vi "UHR-Fleezers Control (host) -Leonardo 04-2018 V3_greenctrl.vi"(0 "Tab Green FB":T5(tab)=enum."Trap Control (RF)") -> ()   [LabVIEW 2013] (continued)
        n482 = property on="APD Chart" class="WFChart (strict)"("YScale.Minimum"=w832) -> ()  [unwired: 2 in, 2 out]
        n483 = property on="APD Chart" class="WFChart (strict)"("YScale.Maximum"=w831) -> ()  [unwired: 2 in, 2 out]
      }
      event "Phase adj. (AI1)", "+ phase (AI1)", "- phase (AI1)": Value Change {
        n484 = event-data() -> ()  [unwired: 7 out]
        n485 = Negate(x="Phase adj. (AI1)") -> (-x=w848:i16)
        n486 = Select(t=w848, s="- phase (AI1)", f="Phase adj. (AI1)") -> (s? t:f=w847:i16)
        n487 = xnode "Read/Write Control"("FPGA VI Reference In"=w851, "error in"=w850, "Phase count adjustment"=w847) -> ("FPGA VI Reference Out"=w846:T20, "error out"=w845:errorcluster)
        n488 = Or(x="- phase (AI1)", y="+ phase (AI1)") -> (x .or. y?=w842:bool)
        n489 = xnode "Read/Write Control"("FPGA VI Reference In"=w846, "error in"=w845, "+ phase"=w842) -> ("error out"=w841:errorcluster)  [unwired: 1 out]
      }
      event "Signals to Plot": Double Click {
        w854 = u32 9868950 ("Color Box")
        n490 = event-data() -> ("Row"=w856:i32)  [unwired: 9 out]
        n491 = property on="All Signals" class="WFChart (strict)"("Active Plot"=w856) -> (error out=w867:errorcluster)  [unwired: 2 in, 1 out]
        n492 = property on="All Signals" class="WFChart (strict)" props=["Plot", "Visible?", "Plot", "Plot Color"](error in=w867) -> (error out=w866:errorcluster, "Plot.Visible?"=w865:bool)  [unwired: 1 in, 2 out]
        n493 = Select(t=FALSE ("Plot.Visible"), s=w865, f=TRUE ("Plot.Visible")) -> (s? t:f=w860:bool)
        n494 = property on="All Signals" class="WFChart (strict)"(error in=w866, "Plot.Visible?"=w860) -> (error out=w862:errorcluster)  [unwired: 1 in, 1 out]
        n495 = property on="All Signals" class="WFChart (strict)"(error in=w862) -> (error out=w857:errorcluster, "Plot.Plot Color"=w861:u32)  [unwired: 1 in, 1 out]
        n496 = property on="Signals to Plot" class="LstBox (strict)"(error in=w857, "Active Row"=w856) -> (error out=w855:errorcluster)  [unwired: 1 in, 1 out]
        n497 = Select(t=w861, s=w860, f=u32 0) -> (s? t:f=w858:u32)
        n498 = property on="Signals to Plot" class="LstBox (strict)"(error in=w855, "CellFontColor"=w858, "SelColor"=w854, "CellBG"=w854, "CellFontSize"=u32 20 ("Active Row:Cell Font:Size"), "CellFontBold"=TRUE ("Active Row:Cell Font:Bold")) -> ()  [unwired: 1 in, 2 out]
      }
      event "Dynamic Force FB": Value Change {
        n499 = event-data() -> ()  [unwired: 7 out]
        n500 = xnode "Read/Write Control"("FPGA VI Reference In"=w869, "Dynamic Force FB (Ronen)"="Dynamic Force FB") -> ()  [unwired: 1 in, 2 out]
      }
      event "BD 1 Frequency 1 (MHz)", "BD 1 Frequency 2 (MHz)", "BD 1 Frequency 3 (MHz)", "BD 2 Frequency 1 (MHz)", "BD 2 Frequency 2 (MHz)", "BD 2 Frequency 3 (MHz)", "Trap Delta (MHz)": Value Change {
        # "anytime one of the frequencies is changed, write it to the RF board UNLESS Set 2 is being oscillated. The oscillation\nscript writes the frequencies to the RF board."
        n501 = event-data() -> ("CtlRef"=w872:refnum<vi>)  [unwired: 6 out]
        n502 = control-ref of="Trap Delta (MHz)"() -> (w871:refnum<vi>)
        n503 = Equal?(x=w871, y=w872) -> (x = y?=w870:bool)
        n504 = case shown="False" "Oscillate Set 2" {
          tunnel: w875 -> [w896 _]
          tunnel: [w895 w908] -> w874
          tunnel: w873 -> [w894 w908]
          tunnel: w870 -> [w881 _]
          frame False {
            n505 = case shown="True" "Symmetric manual \ntrap motion" {
              tunnel: ["T2 for asymmetric\n(MHz)" w907] -> w882
              tunnel: "Trap Delta (MHz)" -> [w901 w906]
              tunnel: [w900 w903] -> w878
              frame False {
                n506 = Subtract(x="T2 for asymmetric\n(MHz)", y=w901) -> (x-y=w900:dbl)
              }
              frame True {
                n507 = Divide(x=w906, y=2) -> (x/y=w904:dbl)
                n508 = Subtract(x="Middle freq for \nsymmetric (MHz)", y=w904) -> (x-y=w903:dbl)
                n509 = Add(x="Middle freq for \nsymmetric (MHz)", y=w904) -> (x+y=w907:dbl)
              }
            }
            n510 = local read "BD 1 Frequency 2 (MHz)"() -> (w883:dbl)
            n511 = local write "BD 1 Frequency 1 (MHz)"(w878) -> ()
            n512 = Select(t=w882, s=w881, f=w883) -> (s? t:f=w880:dbl)
            n513 = local read "Y RF Frequency Limits (MHz)"() -> (w884:T16)
            n514 = local read "X RF Frequency Limits (MHz)"() -> (w885:T16)
            n515 = local read "BD 1 Frequency 3 (MHz)"() -> (w897:dbl)
            n516 = local write "BD 1 Frequency 2 (MHz)"(w880) -> ()
            n517 = local read "BD 2 Frequency 1 (MHz)"() -> (w888:dbl)
            n518 = local read "BD 2 Frequency 2 (MHz)"() -> (w887:dbl)
            n519 = local read "BD 2 Frequency 3 (MHz)"() -> (w898:dbl)
            n520 = call "set RF board frequency - interlace.vi"("Board 2 Frequency Limits"=w884, "Board 1 Frequency Limits"=w885, "error in"=w894, "FPGA VI Reference In"=w896, "Board 2 Frequency 3 (MHz)"=w898, "Board 1 Frequency 3 (MHz)"=w897, "Board 2 Frequency 2 (MHz)"=w887, "Board 2 Frequency 1 (MHz)"=w888, "Board 1 Frequency 2 (MHz)"=w880, "Board 1 Frequency 1  (MHz)"=w878) -> ("error out"=w895:errorcluster)  [unwired: 1 out]
            n521 = Subtract(x=w888, y=w887) -> (x-y=w892:dbl)
            n522 = Subtract(x=w880, y=w878) -> (x-y=w893:dbl)
            n523 = Square(x=w892) -> (x^2=w890:dbl)
            n524 = Square(x=w893) -> (x^2=w891:dbl)
            n525 = Add(x=w891, y=w890) -> (x+y=w889:dbl)
            n526 = Square Root(x=w889) -> (sqrt(x)=w886:dbl)
            n527 = local write "Trap Delta (MHz)"(w886) -> ()
            n528 = property on="Initial delta (MHz)" class="DigNum (strict)"("Val(Sgnl)"=w886) -> ()  [unwired: 2 in, 2 out]
          }
          frame True {
          }
        }
      }
      event "Round T1 X": Value Change {
        n529 = event-data() -> ()  [unwired: 7 out]
        n530 = local read "BD 1 Frequency 1 (MHz)"() -> (w911:dbl)
        n531 = Round To Nearest(number=w911) -> (nearest integer value=w910:dbl)
        n532 = property on="BD 1 Frequency 1 (MHz)" class="DigNum (strict)"("Val(Sgnl)"=w910) -> ()  [unwired: 2 in, 2 out]
      }
      event "Round T2 X": Value Change {
        n533 = event-data() -> ()  [unwired: 7 out]
        n534 = local read "BD 1 Frequency 2 (MHz)"() -> (w913:dbl)
        n535 = Round To Nearest(number=w913) -> (nearest integer value=w912:dbl)
        n536 = property on="BD 1 Frequency 2 (MHz)" class="DigNum (strict)"("Val(Sgnl)"=w912) -> ()  [unwired: 2 in, 2 out]
      }
      event "Stop All": Value Change {
        n537 = event-data() -> ()  [unwired: 7 out]
        n538 = call "hamilton_controller.vi"("action"=T21."DISCONNECT") -> ()  [unwired: 10 in, 1 out]
        n539 = local read "Stop All"() -> (w916:bool)
      }
      event "Delayed Interlace Start": Value Change {
        n540 = event-data() -> ()  [unwired: 7 out]
        n541 = flat-sequence {
          frame #0 {
            n542 = Multiply(x="Delay to Interlace (s)", y=1000.0) -> (x*y=w919:dbl)
            n543 = Wait (ms)(milliseconds to wait=w919) -> ()  [unwired: 1 out]
          }
          frame #1 {
            n544 = property on="Green laser mode" class="RadioBtnsControl (strict)"("Val(Sgnl)"=enum32{"Laser ON", "Laser OFF", "Interlace"}."Interlace" ("Value (Signaling)")) -> ()  [unwired: 2 in, 2 out]
          }
        }
      }
      event "BD 1 Amplitude 1 (%)", "BD 1 Amplitude 2 (%)", "BD 1 Amplitude 3 (%)", "BD 2 Amplitude 1 (%)", "BD 2 Amplitude 2 (%)", "BD 2 Amplitude 3 (%)", "Trap 1 ON", "Trap 2 ON", "Trap 3 ON", "Feedback On/Off", "All FB On/Off": Value Change {
        w943 = i16 1 ("f")
        n545 = event-data() -> ()  [unwired: 7 out]
        n546 = local write "Trap 1 (ON/OFF)"("Trap 1 ON") -> ()
        n547 = local write "Trap 2 (ON/OFF)"("Trap 2 ON") -> ()
        n548 = Boolean To (0,1)(Boolean="Trap 3 ON") -> (0, 1=w944:i16)
        n549 = Boolean To (0,1)(Boolean="Trap 1 ON") -> (0, 1=w945:i16)
        n550 = Boolean To (0,1)(Boolean="Trap 2 ON") -> (0, 1=w946:i16)
        n551 = Select(t=w946, s="Trap ON/OFF X or Y Amp?", f=w943) -> (s? t:f=w941:i16)
        n552 = Select(t=w945, s="Trap ON/OFF X or Y Amp?", f=w943) -> (s? t:f=w942:i16)
        n553 = Select(t=w944, s="Trap ON/OFF X or Y Amp?", f=w943) -> (s? t:f=w940:i16)
        n554 = Select(t=w943, s="Trap ON/OFF X or Y Amp?", f=w946) -> (s? t:f=w938:i16)
        n555 = Select(t=w943, s="Trap ON/OFF X or Y Amp?", f=w945) -> (s? t:f=w939:i16)
        n556 = Select(t=w943, s="Trap ON/OFF X or Y Amp?", f=w944) -> (s? t:f=w937:i16)
        n557 = And(x="All FB On/Off", y="Feedback On/Off") -> (x .and. y?=w935:cluster{"Set 1":bool, "Set 2":bool})
        n558 = local read "BD 1 Amplitude 1 (%)"() -> (w955:dbl)
        n559 = local read "BD 1 Amplitude 2 (%)"() -> (w954:dbl)
        n560 = local read "BD 1 Amplitude 3 (%)"() -> (w953:dbl)
        n561 = Unbundle By Name(w935) -> ("Set 1"=w931:bool, "Set 2"=w928:bool)
        n562 = local read "Y RF Amplitude Limits (%)"() -> (w924:T16)
        n563 = local read "X RF Amplitude Limits (%)"() -> (w925:T16)
        n564 = local read "BD 2 Amplitude 1 (%)"() -> (w956:dbl)
        n565 = local read "BD 2 Amplitude 2 (%)"() -> (w957:dbl)
        n566 = local read "BD 2 Amplitude 3 (%)"() -> (w958:dbl)
        n567 = And(x="Trap 2 ON", y=w928) -> (x .and. y?=w926:bool)
        n568 = And(x="Trap 1 ON", y=w931) -> (x .and. y?=w929:bool)
        n569 = Multiply(x=w942, y=w955) -> (x*y=w950:dbl)
        n570 = Multiply(x=w954, y=w941) -> (x*y=w948:dbl)
        n571 = Multiply(x=w953, y=w940) -> (x*y=w949:dbl)
        n572 = Multiply(x=w956, y=w939) -> (x*y=w959:dbl)
        n573 = Multiply(x=w957, y=w938) -> (x*y=w960:dbl)
        n574 = Multiply(x=w958, y=w937) -> (x*y=w961:dbl)
        n575 = call "set RF board amplitude - interlace.vi"("Board 2 Amplitude Limits"=w924, "Board 1 Amplitude Limits"=w925, "error in"=w951, "FPGA VI Reference In"=w952, "Board 2 Amplitude 3 (%)"=w961, "Board 1 Amplitude 3 (%)"=w949, "Board 2 Amplitude 2 (%)"=w960, "Board 2 Amplitude 1 (%)"=w959, "Board 1 Amplitude 2 (%)"=w948, "Board 1 Amplitude 1 (%)"=w950) -> ("error out"=w933:errorcluster, "FPGA VI Reference Out"=w934:T20)
        n576 = xnode "Read/Write Control"("FPGA VI Reference In"=w934, "error in"=w933, "FB On/Off Set 1"=w929, "FB On/Off Set 2"=w926) -> ("error out"=w932:errorcluster)  [unwired: 1 out]
        n577 = case shown="True" "All FB On/Off" {
          frame False {
          }
          frame True {
            n578 = local write "Feedback overload"(FALSE) -> ()
          }
        }
      }
      event "Load parameters": Value Change {
        n579 = event-data() -> ()  [unwired: 7 out]
        n580 = property on="Saved AOD Raster Scan Parameter Sets" class="Arr (strict)"() -> ("Index Values"=w973:u32[])  [unwired: 2 in, 2 out]
        n581 = Index Array(array=w973, index=0) -> (element=w970:u32)
        n582 = local write "Load parameters"(FALSE ("Load parameters")) -> ()
        n583 = Index Array(array="Saved AOD Raster Scan Parameter Sets", index=w970) -> (element=w969:T31)
        n584 = Unbundle By Name(w969) -> ("Scan Range AOD (nm) 2"=w968:dbl, "Step Size AOD (nm) 2"=w967:dbl, "Scan Speed AOD (nm/s) 2"=w966:dbl, "Number of scans (AOD) 2"=w965:u16)
        n585 = flat-sequence {
          tunnel: w968 -> [w976]
          tunnel: w967 -> [w975]
          tunnel: w966 -> [w974]
          tunnel: w965 -> [w977]
          frame #0 {
            n586 = local write "Scan Speed (nm/s)"(w974) -> ()
            n587 = local write "Scan Range (nm)"(w976) -> ()
            n588 = local write "Step Size (nm)"(w975) -> ()
          }
          frame #1 {
            n589 = property on="Number of F/B Scans (AOD)" class="DigNum (strict)"("Val(Sgnl)"=w977) -> ()  [unwired: 2 in, 2 out]
          }
        }
      }
      event "Trap 1 (ON/OFF)", "Trap 2 (ON/OFF)": Value Change {
        n590 = event-data() -> ()  [unwired: 7 out]
        n591 = property on="Trap 2 ON" class="Bool (strict)"("Val(Sgnl)"="Trap 2 (ON/OFF)") -> ()  [unwired: 2 in, 2 out]
        n592 = property on="Trap 1 ON" class="Bool (strict)"("Val(Sgnl)"="Trap 1 (ON/OFF)") -> ()  [unwired: 2 in, 2 out]
      }
      event "DIO count 1 (ticks)", "DIO count 2 (ticks)", "DIO count 3 (ticks)", "Interlace", "Number Interlace Sets", "Not-Interlacing Set": Value Change {
        n593 = event-data() -> ()  [unwired: 7 out]
        n594 = local read "DIO count 3 (ticks)"() -> (w990:u32)
        n595 = local read "DIO count 1 (ticks)"() -> (w992:u32)
        n596 = local read "DIO count 2 (ticks)"() -> (w991:u32)
        n597 = To Unsigned Byte Integer(number="Not-Interlacing Set") -> (unsigned 8bit integer=w981:u8)
        n598 = Add(x=w981, y=u8 1) -> (x+y=w985:u8)
        n599 = xnode "Read/Write Control"("FPGA VI Reference In"=w996, "error in"=w994, "DIO count 1 (ticks)"=w992, "DIO count 2 (ticks)"=w991, "DIO count 3 (ticks)"=w990, "Interlace ON/OFF"="Interlace", "Number Interlace Cycles"="Number Interlace Sets", "Interlace Off Parameters"=w985) -> ("error out"=w995:errorcluster)  [unwired: 1 out]
        n600 = Build Array(w992, w991, w990) -> (w983:u32[])
        n601 = Split 1D Array(array=w983, index="Number Interlace Sets") -> (first subarray=w993:u32[])  [unwired: 1 out]
        n602 = Index Array(array=w983, index=w981) -> (element=w982:u32)
        n603 = Add Array Elements(numeric array=w993) -> (sum=w987:u32)
        n604 = Select(t=w987, s="Interlace", f=w982) -> (s? t:f=→"Total Counts (ticks)":u32)
      }
      event "Reset Feedback": Value Change {
        n605 = event-data() -> ()  [unwired: 7 out]
        n606 = Unbundle By Name("Reset Feedback") -> ("Set 1"=w1000:bool, "Set 2"=w999:bool)
        n607 = xnode "Read/Write Control"("FPGA VI Reference In"=w1002, "error in"=w997, "FB Reset Set 1"=w1000, "FB Reset Set 2"=w999) -> ("error out"=w998:errorcluster)  [unwired: 1 out]
      }
      event "PID gains": Value Change {
        n608 = event-data() -> ()  [unwired: 7 out]
        n609 = local read "PID gains"() -> (w1003:T10)
        n610 = xnode "Read/Write Control"("FPGA VI Reference In"=w1006, "error in"=w1004, "FB Gains"=w1003) -> ("error out"=w1005:errorcluster)  [unwired: 1 out]
      }
      event "AI2 to Setpoint", "Trap Intensity\nSetpoints (V)": Value Change {
        n611 = event-data() -> ()  [unwired: 7 out]
        n612 = xnode "Read/Write Control"("FPGA VI Reference In"=w1011, "error in"=w1007) -> ("FPGA VI Reference Out"=w1010:T20, "error out"=w1009:errorcluster, "AI2 Y Sum Set 1"=w1018:i16, "AI2 Y Sum Set 2"=w1017:i16)
        n613 = Cluster To Array(cluster="AI2 to Setpoint") -> (array=w1021:bool[])
        n614 = local read "AI2 (V)"() -> (w1019:cluster{"Set 1":dbl, "Set 2":dbl})
        n615 = Or Array Elements(Boolean array=w1021) -> (logical OR=w1022:bool)
        n616 = Bundle By Name(cluster=w1019, "Set 1"=w1018, "Set 2"=w1017) -> (w1016:cluster{"Set 1":dbl, "Set 2":dbl})
        n617 = Divide(x=w1016, y=3276.7) -> (x/y=w1015:cluster{"Set 1":dbl, "Set 2":dbl})
        "AI2 (V)" <- w1015
        n618 = case shown="True" w1022 {
          tunnel: [w1025 w1042] -> w1014
          tunnel: "AI2 to Setpoint" -> [_ w1038]
          tunnel: "Trap Intensity\nSetpoints (V)" -> [w1026 w1041]
          tunnel: w1015 -> [_ w1035]
          frame False {
            n619 = Multiply(x=3276.7, y=w1026) -> (x*y=w1027:cluster{"Set 1":dbl, "Set 2":dbl})
            n620 = To Word Integer(number=w1027) -> (16bit integer=w1025:cluster{"Set 1":i16, "Set 2":i16})
          }
          frame True {
            n621 = Unbundle By Name(w1035) -> ("Set 1"=w1034:dbl, "Set 2"=w1033:dbl)
            n622 = Unbundle By Name(w1041) -> ("Set 1"=w1040:dbl, "Set 2"=w1039:dbl)
            n623 = Unbundle By Name(w1038) -> ("Set 1"=w1037:bool, "Set 2"=w1036:bool)
            n624 = Select(t=w1034, s=w1037, f=w1040) -> (s? t:f=w1032:dbl)
            n625 = Select(t=w1033, s=w1036, f=w1039) -> (s? t:f=w1031:dbl)
            n626 = Bundle By Name(cluster=w1041, "Set 1"=w1032, "Set 2"=w1031) -> (w1029:cluster{"Set 1":dbl, "Set 2":dbl})
            n627 = local write "Trap Intensity\nSetpoints (V)"(w1029) -> ()
            n628 = Multiply(x=3276.7, y=w1029) -> (x*y=w1030:cluster{"Set 1":dbl, "Set 2":dbl})
            n629 = To Word Integer(number=w1030) -> (16bit integer=w1042:cluster{"Set 1":i16, "Set 2":i16})
          }
        }
        n630 = Unbundle By Name(w1014) -> ("Set 1"=w1013:i16, "Set 2"=w1012:i16)
        n631 = xnode "Read/Write Control"("FPGA VI Reference In"=w1010, "error in"=w1009, "FB Setpoint Set 1"=w1013, "FB Setpoint Set 2"=w1012) -> ("error out"=w1008:errorcluster)  [unwired: 1 out]
      }
      event "Invert GI": Value Change {
        n632 = event-data() -> ()  [unwired: 7 out]
        n633 = xnode "Read/Write Control"("FPGA VI Reference In"=w1047, "error in"=w1045, "Invert GI"="Invert GI", "Invert GI 2"="Invert GI") -> ("error out"=w1046:errorcluster)  [unwired: 1 out]
      }
      event "Green FB Setpoint (mV)", "Green FB Gains", "Green FB On/Off", "Current When FB OFF (%)", "Green int current ON count adj": Value Change {
        n634 = event-data() -> ()  [unwired: 7 out]
        n635 = local read "Green FB Setpoint (mV)"() -> (w1054:dbl)
        n636 = local read "Current When FB OFF (%)"() -> (w1057:dbl)
        n637 = Multiply(x=w1054, y=3.2767) -> (x*y=w1053:dbl)
        n638 = Multiply(x=w1057, y=655.35) -> (x*y=w1058:dbl)
        n639 = To Unsigned Word Integer(number=w1058) -> (unsigned 16bit integer=w1056:u16)
        n640 = local read "Green int current ON count adj"() -> (w1061:u32)
        n641 = local read "Green FB Gains"() -> (w1060:T10)
        n642 = local read "Green Laser ON/Interlacing"() -> (w1051:bool)
        n643 = local read "Green laser mode"() -> (w1050:enum32{"Laser ON", "Laser OFF", "Interlace"})
        n644 = local read "Green FB On/Off"() -> (w1062:bool)
        n645 = Equal?(x=w1050, y=enum32{"Laser ON", "Laser OFF", "Interlace"}."Interlace") -> (x = y?=w1048:bool)
        n646 = Compound Arithmetic op=AND(w1048, w1062, w1051) -> (w1052:bool)
        n647 = xnode "Read/Write Control"("FPGA VI Reference In"=w1065, "error in"=w1064, "Green FB Setpoint"=w1053, "Green FB On/Off"=w1052, "Current Out"=w1056, "Green int current ON count adj"=w1061, "Green FB Gains"=w1060) -> ("error out"=w1063:errorcluster)  [unwired: 1 out]
      }
      event "Green laser mode", "Green Laser ON/Interlacing": Value Change {
        n648 = event-data() -> ()  [unwired: 7 out]
        n649 = case shown="True" "Green Laser ON/Interlacing" {
          tunnel: "Green laser mode" -> [_ w1079]
          tunnel: [enum32{"Laser ON", "Laser OFF", "Interlace"}."Laser OFF" ("Green laser mode") w1079] -> w1067
          tunnel: [FALSE w1075] -> w1066
          frame False {
          }
          frame True {
            n650 = local read "Green FB On/Off"() -> (w1076:bool)
            n651 = Equal?(x=w1079, y=enum32{"Laser ON", "Laser OFF", "Interlace"}."Interlace") -> (x = y?=w1077:bool)
            n652 = And(x=w1077, y=w1076) -> (x .and. y?=w1075:bool)
          }
        }
        n653 = xnode "Read/Write Control"("FPGA VI Reference In"=w1072, "error in"=w1070, "Operating Mode"=w1067, "Operating Mode 2"=w1067, "Green FB On/Off"=w1066) -> ("error out"=w1071:errorcluster)  [unwired: 1 out]
      }
      event "- phase (APD 1 Gate)", "+ phase (APD 1 Gate)": Value Change {
        n654 = event-data() -> ()  [unwired: 7 out]
        n655 = local read "Phase Adj. (APD 1 Gate)"() -> (w1080:i16)
        n656 = Negate(x=w1080) -> (-x=w1088:i16)
        n657 = Select(t=w1088, s="- phase (APD 1 Gate)", f=w1080) -> (s? t:f=w1087:i16)
        n658 = Or(x="- phase (APD 1 Gate)", y="+ phase (APD 1 Gate)") -> (x .or. y?=w1083:bool)
        n659 = xnode "Read/Write Control"("FPGA VI Reference In"=w1090, "error in"=w1089, "Phase count adjustment (APD 1 Gate)"=w1087) -> ("FPGA VI Reference Out"=w1085:T20, "error out"=w1086:errorcluster)
        n660 = xnode "Read/Write Control"("FPGA VI Reference In"=w1085, "error in"=w1086, "+ phase (APD 1 Gate)"=w1083) -> ("error out"=w1084:errorcluster)  [unwired: 1 out]
      }
      event "+ phase (APD 2 Gate)", "- phase (APD 2 Gate)": Value Change {
        n661 = event-data() -> ()  [unwired: 7 out]
        n662 = local read "Phase Adj. (APD 2 Gate)"() -> (w1091:i16)
        n663 = Negate(x=w1091) -> (-x=w1099:i16)
        n664 = Select(t=w1099, s="- phase (APD 2 Gate)", f=w1091) -> (s? t:f=w1098:i16)
        n665 = Or(x="- phase (APD 2 Gate)", y="+ phase (APD 2 Gate)") -> (x .or. y?=w1094:bool)
        n666 = xnode "Read/Write Control"("FPGA VI Reference In"=w1101, "error in"=w1100, "Phase count adjustment (APD 2 Gate)"=w1098) -> ("FPGA VI Reference Out"=w1096:T20, "error out"=w1097:errorcluster)
        n667 = xnode "Read/Write Control"("FPGA VI Reference In"=w1096, "error in"=w1097, "+ phase (APD 2 Gate)"=w1094) -> ("error out"=w1095:errorcluster)  [unwired: 1 out]
      }
      event "Phase Adj. (APD Acq)", "+ phase (APD Acq)", "- phase (APD Acq)": Value Change {
        n668 = event-data() -> ()  [unwired: 7 out]
        n669 = local read "Phase Adj. (APD Acq)"() -> (w1104:i16)
        n670 = Negate(x=w1104) -> (-x=w1110:i16)
        n671 = Select(t=w1110, s="+ phase (APD Acq)", f=w1104) -> (s? t:f=w1109:i16)
        n672 = Or(x="+ phase (APD Acq)", y="- phase (APD Acq)") -> (x .or. y?=w1105:bool)
        n673 = xnode "Read/Write Control"("FPGA VI Reference In"=w1112, "error in"=w1111, "Phase Count Adjustment (APD Acq)"=w1109) -> ("FPGA VI Reference Out"=w1107:T20, "error out"=w1108:errorcluster)
        n674 = xnode "Read/Write Control"("FPGA VI Reference In"=w1107, "error in"=w1108, "+ phase (APD Acq)"=w1105) -> ("error out"=w1106:errorcluster)  [unwired: 1 out]
      }
      event "Phase adj. (GI)", "+ phase (GI)", "- phase (GI)": Value Change {
        n675 = event-data() -> ()  [unwired: 7 out]
        n676 = Negate(x="Phase adj. (GI)") -> (-x=w1121:i16)
        n677 = Select(t=w1121, s="+ phase (GI)", f="Phase adj. (GI)") -> (s? t:f=w1120:i16)
        n678 = Or(x="+ phase (GI)", y="- phase (GI)") -> (x .or. y?=w1116:bool)
        n679 = xnode "Read/Write Control"("FPGA VI Reference In"=w1123, "error in"=w1122, "Phase count adjustment (GI)"=w1120) -> ("FPGA VI Reference Out"=w1118:T20, "error out"=w1119:errorcluster)
        n680 = xnode "Read/Write Control"("FPGA VI Reference In"=w1118, "error in"=w1119, "+ phase (GI)"=w1116) -> ("error out"=w1117:errorcluster)  [unwired: 1 out]
      }
      event "Phase adj. (GI) 2", "+ phase (GI) 2", "- phase (GI) 2": Value Change {
        n681 = event-data() -> ()  [unwired: 7 out]
        n682 = Negate(x="Phase adj. (GI) 2") -> (-x=w1132:i16)
        n683 = Select(t=w1132, s="+ phase (GI) 2", f="Phase adj. (GI) 2") -> (s? t:f=w1131:i16)
        n684 = Or(x="+ phase (GI) 2", y="- phase (GI) 2") -> (x .or. y?=w1127:bool)
        n685 = xnode "Read/Write Control"("FPGA VI Reference In"=w1134, "error in"=w1133, "Phase count adjustment (GI) 2"=w1131) -> ("FPGA VI Reference Out"=w1129:T20, "error out"=w1130:errorcluster)
        n686 = xnode "Read/Write Control"("FPGA VI Reference In"=w1129, "error in"=w1130, "+ phase (GI) 2"=w1127) -> ("error out"=w1128:errorcluster)  [unwired: 1 out]
      }
      event "Phase adj. (Green FB)", "- phase (Green FB)", "+ phase (Green FB)": Value Change {
        n687 = event-data() -> ()  [unwired: 7 out]
        n688 = Negate(x="Phase adj. (Green FB)") -> (-x=w1143:i16)
        n689 = Select(t=w1143, s="+ phase (Green FB)", f="Phase adj. (Green FB)") -> (s? t:f=w1142:i16)
        n690 = Or(x="+ phase (Green FB)", y="- phase (Green FB)") -> (x .or. y?=w1138:bool)
        n691 = xnode "Read/Write Control"("FPGA VI Reference In"=w1145, "error in"=w1144, "Phase count adjustment (Green FB)"=w1142) -> ("FPGA VI Reference Out"=w1140:T20, "error out"=w1141:errorcluster)
        n692 = xnode "Read/Write Control"("FPGA VI Reference In"=w1140, "error in"=w1141, "+ phase (Green FB)"=w1138) -> ("error out"=w1139:errorcluster)  [unwired: 1 out]
      }
      event "Invert APD Gate", "APD Gate ON Count", "APD Gate OFF Count", "APD Gate", "APD Integration Time (s)", "APD 1 AO Mult.", "APD 2 AO Mult.": Value Change {
        n693 = event-data() -> ()  [unwired: 7 out]
        n694 = local read "APD Integration Time (s)"() -> (w1146:dbl)
        n695 = local read "APD Gate ON Count"() -> (w1159:u32)
        n696 = local read "APD Gate OFF Count"() -> (w1158:u32)
        n697 = local read "Invert APD Gate"() -> (w1160:bool)
        n698 = local read "APD Gate"() -> (w1157:enum32{"ON", "OFF", "Interlace"})
        n699 = Multiply(x=w1146, y=40000000.0) -> (x*y=w1155:dbl)
        n700 = Reciprocal(x=w1146) -> (1/x=→"APD Acq Rate (Hz)":dbl)
        n701 = To Unsigned Long Integer(number=w1155) -> (unsigned 32bit integer=w1154:u32)
        n702 = local read "DMA Update Period (s)"() -> (w1147:dbl)
        n703 = Divide(x=w1147, y=w1146) -> (x/y=w1150:dbl)
        n704 = local read "APD 1 AO Mult."() -> (w1152:i16)
        n705 = local read "APD 2 AO Mult."() -> (w1151:i16)
        n706 = Multiply(x=2.0, y=w1150) -> (x*y=w1149:dbl)
        n707 = local write "APD Samples/FIFO Acq."(w1150) -> ()
        n708 = local write "APD Elements/DMA read"(w1149) -> ()
        n709 = xnode "Read/Write Control"("FPGA VI Reference In"=w1163, "error in"=w1162, "Invert APD Gate"=w1160, "APD Gate ON Count"=w1159, "APD Gate OFF Count"=w1158, "APD Acq Rate Count"=w1154, "APD Gate Operating Mode"=w1157, "APD 1 AO scale factor"=w1152, "APD 2 AO scale factor"=w1151) -> ("error out"=w1161:errorcluster)  [unwired: 1 out]
      }
      event "GI Frequency, ON count", "Green FB Count", "GI Frequency, OFF count": Value Change {
        n710 = event-data() -> ()  [unwired: 7 out]
        n711 = xnode "Read/Write Control"("FPGA VI Reference In"=w1169, "error in"=w1167, "Green interlace ON count"="GI Frequency, ON count", "Green interlace OFF count"="GI Frequency, OFF count", "Green interlace ON count 2"="GI Frequency, ON count", "Green interlace OFF count 2"="GI Frequency, OFF count", "Green FB Count"="Green FB Count") -> ("error out"=w1168:errorcluster)  [unwired: 1 out]
      }
      event "Number of F/B Scans (AOD)", "Scan Speed (nm/s)", "Scan BD", "Initial delta (MHz)", "Step Size (nm)", "Scan Range (nm)": Value Change {
        w1231 = 123.0  # AOM cal (nm/MHz)
        n712 = event-data() -> ()  [unwired: 7 out]
        n713 = local read "BD 1 Frequency 1 (MHz)"() -> (w1214:dbl)
        n714 = local read "AOM X Cal (nm/MHz)"() -> (w1206:dbl)
        n715 = local read "X RF Frequency Limits (MHz)"() -> (w1218:T16)
        n716 = local read "Y RF Frequency Limits (MHz)"() -> (w1215:T16)
        n717 = local read "BD 2 Frequency 1 (MHz)"() -> (w1220:dbl)
        n718 = Negate(x="Scan Range (nm)") -> (-x=w1184:dbl)
        n719 = Divide(x=w1184, y=w1206) -> (x/y=w1188:dbl)
        n720 = Select(t=w1218, s="Scan BD", f=w1215) -> (s? t:f=w1217:T16)
        n721 = Select(t=w1214, s="Scan BD", f=w1220) -> (s? t:f=w1219:dbl)
        n722 = Unbundle By Name(w1217) -> ("Maximum"=w1226:dbl, "Minimum"=w1225:dbl)
        n723 = Add(x=w1188, y=w1219) -> (x+y=w1223:dbl)
        n724 = Divide(x=w1184, y="Step Size (nm)") -> (x/y=w1203:dbl)
        n725 = Divide(x="Step Size (nm)", y=w1206) -> (x/y=w1212:dbl)
        n726 = Absolute Value(x=w1203) -> (abs(x)=w1187:dbl)
        n727 = Sign(1:w1184) -> (0:w1185:dbl)
        n728 = In Range and Coerce(upper limit=w1226, x=w1223, lower limit=w1225) -> (coerced(x)=w1222:dbl, In Range?=w1224:bool)
        n729 = To Unsigned Quad Integer(1:w1187) -> (0:w1202:u64)
        "Scan steps (AOD)" <- w1202
        n730 = call "IR AOM freq to word.vi"("Frequency In (MHz)"=w1212) -> ("Frequency Word Out (double)"=w1209:dbl)
        n731 = Multiply(x=w1185, y=w1209) -> (x*y=w1186:dbl)
        n732 = Subtract(x=w1223, y=w1222) -> (x-y=w1221:dbl)
        n733 = To Quad Integer(1:w1186) -> (0:w1208:i64)
        "Incr. int (AOD)" <- w1208
        n734 = Subtract(x=w1188, y=w1221) -> (x-y=w1207:dbl)
        "Scan Range (MHz)" <- w1207
        n735 = Select(t=w1188, s=w1224, f=w1207) -> (s? t:f=w1227:dbl)
        n736 = Multiply(x=w1207, y=w1206) -> (x*y=w1205:dbl)
        n737 = Decrement(x=w1202) -> (x-1=w1255:u64)
        n738 = Negate(x=w1205) -> (-x=w1201:dbl)
        n739 = local write "Scan Range (nm)"(w1201) -> ()
        n740 = Divide(x=w1227, y=w1255) -> (x/y=w1211:dbl)
        "Scan Increment (MHz)" <- w1211
        n741 = call "IR AOM freq to word.vi"("Frequency In (MHz)"=w1211) -> ("Frequency Word Out (double)"=w1210:dbl)
        n742 = Divide(x="Step Size (nm)", y="Scan Speed (nm/s)") -> (x/y=w1198:dbl)
        n743 = To Quad Integer(1:w1210) -> ()  [unwired: 1 out]
        n744 = local read "Number Interlace Sets"() -> (w1182:u8)
        n745 = local read "AI Count (ticks)"() -> (w1183:u32)
        n746 = local read "Total Counts (ticks)"() -> (w1181:u32)
        n747 = local read "# Samples/trap"() -> (w1213:u32)
        n748 = Multiply(x=w1183, y=w1182) -> (x*y=w1180:u32)
        n749 = Divide(x=w1181, y=w1180) -> (x/y=w1179:dbl)
        n750 = Select(t=w1214, s="Scan BD", f=w1220) -> (s? t:f=w1252:dbl)
        "Initial freq. (MHz)" <- w1252
        n751 = Add(x=w1227, y=w1252) -> (x+y=→"Final freq. (MHz)":dbl)
        n752 = Divide(x=w1181, y=40000000.0) -> (x/y=w1197:dbl)
        n753 = Divide(x=w1198, y=w1197) -> (x/y=w1196:dbl)
        n754 = To Unsigned Quad Integer(1:w1196) -> (0:w1171:u64)
        n755 = Quotient & Remainder(x=w1171, y=u64 2) -> (x-y*floor(x/y)=w1175:u64)  [unwired: 1 out]
        n756 = Equal?(x=w1175, y=u64 0) -> (x = y?=w1173:bool)
        n757 = Decrement(x=w1171) -> (x-1=w1172:u64)
        n758 = Select(t=w1171, s=w1173, f=w1172) -> (s? t:f=w1170:u64)
        "Cycles/step (AOD)" <- w1170
        n759 = xnode "Read/Write Control"("FPGA VI Reference In"=w1263, "error in"=w1262, "Scan steps"=w1202, "Number of scans"="Number of F/B Scans (AOD)", "Cycles per step"=w1170, "Scan freq.  increment"=w1208, "Scan BD"="Scan BD") -> ("error out"=w1261:errorcluster)  [unwired: 1 out]
        n760 = Multiply(x=w1202, y=w1170) -> (x*y=w1256:u64)
        n761 = Multiply(x=w1256, y=u64 2) -> (x*y=w1178:u64)
        n762 = Multiply(x=w1179, y=w1178) -> (x*y=w1177:dbl)
        "Data points/scan (f/b)" <- w1177
        n763 = Multiply(x=w1177, y="Number of F/B Scans (AOD)") -> (x*y=w1259:dbl)
        "Data points/scans" <- w1259
        n764 = Divide(x=w1259, y=w1213) -> (x/y=→"N sets should be saved":dbl)
        n765 = Multiply(x=w1256, y=w1197) -> (x*y=w1195:dbl)
        "Time/Scan (s) (AOD)" <- w1195
        n766 = Select(t=w1227, s="Scan BD", f=0.0) -> (s? t:f=w1253:dbl)
        n767 = Select(t=0.0, s="Scan BD", f=w1227) -> (s? t:f=w1249:dbl)
        n768 = local read "BD 2 Frequency 2 (MHz)"() -> (w1245:dbl)
        n769 = local read "BD 1 Frequency 2 (MHz)"() -> (w1248:dbl)
        n770 = Add(x=w1249, y=w1220) -> (x+y=w1246:dbl)
        n771 = Add(x=w1214, y=w1253) -> (x+y=w1247:dbl)
        n772 = Multiply(x=w1195, y=2.0) -> (x*y=w1194:dbl)
        n773 = Multiply(x=w1194, y="Number of F/B Scans (AOD)") -> (x*y=w1191:dbl)
        n774 = Divide(x=w1191, y=60.0) -> (x/y=→"Time to Finish All (min)":dbl)
        n775 = Add(x="Trap 2 Bead Size (nm)", y="Trap 1 Bead Size (nm)") -> (x+y=w1235:dbl)
        n776 = local read "Initial delta (MHz)"() -> (w1232:dbl)
        n777 = Divide(x=w1235, y=2.0) -> (x/y=w1229:dbl)
        n778 = Subtract(x=w1246, y=w1245) -> (x-y=w1243:dbl)
        n779 = Subtract(x=w1247, y=w1248) -> (x-y=w1244:dbl)
        n780 = Square(x=w1243) -> (x^2=w1242:dbl)
        n781 = Square(x=w1244) -> (x^2=w1241:dbl)
        n782 = Add(x=w1241, y=w1242) -> (x+y=w1240:dbl)
        n783 = Square Root(x=w1240) -> (sqrt(x)=w1239:dbl)
        "Final delta (MHz)" <- w1239
        n784 = Multiply(x=w1231, y=w1239) -> (x*y=w1238:dbl)
        n785 = Multiply(x=w1232, y=w1231) -> (x*y=w1230:dbl)
        n786 = Subtract(x=w1230, y=w1229) -> (x-y=→"Initial sep (nm)":dbl)
        n787 = Subtract(x=w1238, y=w1229) -> (x-y=→"Final sep (nm)":dbl)
      }
      event "Raster Scanning...": Value Change {
        n788 = event-data() -> ("NewVal"=w1264:bool)  [unwired: 6 out]
        n789 = case shown="True" w1264 {
          frame False {
          }
          frame True {
            n790 = property on="BD 1 Frequency 1 (MHz)" class="DigNum (strict)"("Val(Sgnl)"=65.0 ("Value (Signaling)")) -> ()  [unwired: 2 in, 2 out]
          }
        }
      }
      event "Phase increment trap 1", "Swap F1 and F2", "Freq switch delay", "Amp switch delay", "Phase increment trap 2", "RF phase reset before cycles", "Phase offset method": Value Change {
        n791 = event-data() -> ()  [unwired: 7 out]
        n792 = local read "Amp switch delay"() -> (w1270:u16)
        n793 = local read "Phase increment trap 1"() -> (w1269:fxp<+/-,64,32>)
        n794 = local read "Freq switch delay"() -> (w1272:u16)
        n795 = local read "Phase increment trap 2"() -> (w1268:fxp<+/-,64,32>)
        n796 = local read "RF phase reset before cycles"() -> (w1267:bool)
        n797 = local read "Swap F1 and F2"() -> (w1271:bool)
        n798 = local read "Phase offset method"() -> (w1266:u8)
        n799 = xnode "Read/Write Control"("FPGA VI Reference In"=w1275, "error in"=w1274, "BD 1 Delay (ticks)"=w1272, "Swap F1 and F2"=w1271, "Amp switch delay"=w1270, "Phase Trap 1"=w1269, "Phase Trap 2"=w1268, "RF phase reset before cycles"=w1267, "Phase offset method"=w1266) -> ("error out"=w1273:errorcluster)  [unwired: 1 out]
      }
      event "Scan steps (MCL)", "Number of scans (MCL)", "Scan Range (V)\n(of steps)", "2D or 1D Scan", "N APD Samp/step", "Fast Scan Dir", "Continuous MCL Scanning", "Scan lines (y)": Value Change {
        w1277 = 32767.0 ("y")
        n800 = event-data() -> ()  [unwired: 7 out]
        n801 = Select(t="Scan lines (y)", s="2D or 1D Scan", f="Number of scans (MCL)") -> (s? t:f=w1282:u64)
        n802 = Decrement(x="Scan steps (MCL)") -> (x-1=w1298:u64)
        n803 = Divide(x="Scan Range (V)\n(of steps)", y=w1298) -> (x/y=w1297:dbl)
        "Desired Scan Incr (V)" <- w1297
        n804 = local read "APD Integration Time (s)"() -> (w1290:dbl)
        n805 = Multiply(x=w1297, y=w1277) -> (x*y=w1306:dbl)
        n806 = Divide(x=w1306, y=10.0) -> (x/y=w1296:dbl)
        "Desired incr (int)" <- w1296
        n807 = local read "Update Count (MCL)"() -> (w1302:u32)
        n808 = Round Toward -Infinity(1:w1296) -> (0:w1305:dbl)
        n809 = To Word Integer(number=w1305) -> (16bit integer=w1280:i16)
        "Actual Incr. int (MCL)" <- w1280
        n810 = Multiply(x=w1290, y=40000000.0) -> (x*y=w1303:dbl)
        n811 = Divide(x=w1303, y=w1302) -> (x/y=w1301:dbl)
        n812 = Multiply(x=i16 10, y=w1280) -> (x*y=w1278:i16)
        n813 = Multiply(x="N APD Samp/step", y=w1301) -> (x*y=w1300:dbl)
        "Cycles/step (MCL)" <- w1300
        n814 = Divide(x=w1278, y=w1277) -> (x/y=→"Actual MCL Inc (V)":dbl)
        n815 = Multiply(x="N APD Samp/step", y="Scan steps (MCL)") -> (x*y=w1292:dbl)
        n816 = local read "APD Samples/FIFO Acq."() -> (w1289:dbl)
        n817 = Multiply(x=w1292, y=u64 2) -> (x*y=w1291:dbl)
        "Data points/scan (f+b)" <- w1291
        n818 = Multiply(x=w1291, y=w1282) -> (x*y=w1309:dbl)
        "Data points/scans (MCL)" <- w1309
        n819 = Multiply(x=w1290, y=w1291) -> (x*y=w1283:dbl)
        "Time/f+b scan (s) (MCL)" <- w1283
        n820 = Divide(x=w1309, y=w1289) -> (x/y=→"N sets should be saved (MCL)":dbl)
        n821 = Multiply(x=w1283, y=w1282) -> (x*y=→"Total Time (s)":dbl)
        n822 = Not(x="Fast Scan Dir") -> (.not. x?=w1287:bool)
        n823 = xnode "Read/Write Control"("FPGA VI Reference In"=w1313, "error in"=w1312, "Scan steps (MCL)"="Scan steps (MCL)", "Number of scans (MCL)"=w1282, "Cycles per step (MCL)"=w1300, "Scan freq.  increment (MCL)"=w1280, "1D or 2D Scan?"="2D or 1D Scan", "MCL Scan Axis"=w1287, "Cont. Scan (MCL)"="Continuous MCL Scanning") -> ("error out"=w1311:errorcluster)  [unwired: 1 out]
      }
      event "Read Cal": Value Change {
        w1350 = 1000.0 ("y")
        w1338 = T30."big-endian, network order" ("byte order (0:big-endian, network order)")
        w1339 = -1 ("count (1)")
        n824 = event-data() -> ()  [unwired: 7 out]
        n825 = local read "Save file name"() -> (w1368:path)
        n826 = local write "Read Cal"(FALSE ("Read Cal")) -> ()
        n827 = Strip Path(path=w1368) -> (stripped path=w1367:path)  [unwired: 1 out]
        n828 = Path To String(path=w1367) -> (string=w1348:string)
        n829 = Concatenate Strings(w1348, "\\current.off" ("string")) -> (w1346:string)
        n830 = Concatenate Strings(w1348, "\\current.cal" ("string")) -> (w1365:string)
        n831 = local read "Scale intensities"() -> (w1318:bool)
        n832 = String To Path(string=w1365) -> (path=w1364:path)
        n833 = String To Path(string=w1346) -> (path=w1345:path)
        n834 = Open/Create/Replace File(file path (use dialog)=w1364, operation (0:open)=T24."open", access (0:read/write)=enum16{"read/write", "read-only", "write-only"}."read-only") -> (refnum out=w1371:refnum<file>, error out=w1360:errorcluster)  [unwired: 1 in, 3 out]
        n835 = Deny Access(4:w1360, 7:w1371) -> (0:w1359:errorcluster, 3:w1363:refnum<file>)  [unwired: 1 out]
        n836 = Open/Create/Replace File(file path (use dialog)=w1345, operation (0:open)=T24."open", access (0:read/write)=enum16{"read/write", "read-only", "write-only"}."read-only") -> (refnum out=w1342:refnum<file>)  [unwired: 1 in, 4 out]
        n837 = Deny Access(7:w1342) -> (3:w1340:refnum<file>)  [unwired: 1 in, 2 out]
        n838 = Read from Binary File(5:0.0, 8:w1359, 9:w1338, 10:w1339, 11:w1363) -> (0:w1358:errorcluster, 2:w1356:dbl[], 3:w1361:refnum<file>)  [unwired: 2 out]
        n839 = Array To Cluster(array=w1356) -> (cluster=w1355:T32)
        n840 = Unbundle(w1355) -> ("[0]"=w1329:dbl, "[1]"=w1328:dbl, "[2]"=w1315:dbl, "[3]"=w1317:dbl, "[4]"=w1354:dbl, "[5]"=w1353:dbl)
        n841 = case "Cal is OK if you load a cal with scale intensities on - Alex 081418" shown="True" w1318 {
          tunnel: w1317 -> [w1373 w1376]
          tunnel: [w1373 w1375] -> w1316
          tunnel: w1315 -> [w1372 w1378]
          tunnel: [w1372 w1377] -> w1314
          frame False {
          }
          frame True {
            n842 = local read "Scale factor"() -> (w1374:dbl)
            n843 = Multiply(x=w1376, y=w1374) -> (x*y=w1375:dbl)
            n844 = Multiply(x=w1378, y=w1374) -> (x*y=w1377:dbl)
          }
        }
        n845 = Close File(refnum=w1361, error in=w1358) -> (error out=→"Read cal error":errorcluster)  [unwired: 1 out]
        n846 = Multiply(x=w1353, y=w1350) -> (x*y=w1351:dbl)
        n847 = local write "T2 kappa_x (pN/nm)"(w1316) -> ()
        n848 = local write "T1 kappa_x (pN/nm)"(w1314) -> ()
        n849 = local write "T1 alpha_x (nm/V)"(w1329) -> ()
        n850 = local write "T2 alpha_x (nm/V)"(w1328) -> ()
        n851 = Read from Binary File(5:0.0, 9:w1338, 10:w1339, 11:w1340) -> (2:w1334:dbl[], 3:w1337:refnum<file>)  [unwired: 1 in, 3 out]
        n852 = Multiply(x=w1354, y=w1350) -> (x*y=w1352:dbl)
        n853 = local write "T1 offset_x (mV)"(w1352) -> ()
        n854 = local write "T2 offset_x (mV)"(w1351) -> ()
        n855 = Close File(refnum=w1337) -> ()  [unwired: 1 in, 2 out]
        n856 = Array Subset(array=w1334, index=3) -> (w1332:dbl[])  [unwired: 1 in]
        n857 = Index Array(array=w1334, index=0) -> (element=→"Offset file step size":dbl)
        n858 = Multiply(x=w1329, y=w1315) -> (x*y=w1326:dbl)
        n859 = Multiply(x=w1328, y=w1317) -> (x*y=w1327:dbl)
        n860 = Divide(x=w1327, y=w1326) -> (x/y=w1320:dbl)
        n861 = Decimate 1D Array(w1332) -> (w1324:dbl[], w1325:dbl[])  [unwired: 1 out]
        n862 = disable-structure "Removed B factor to improve position FB -Alex 081418 2of3" shown="Enabled" {
          disable-tunnel: w1320 -> [w1379 _]
          disable-tunnel: [w1379 1.0] -> w1319
          frame Disabled {
          }
          frame Enabled {
          }
        }
        n863 = Bundle By Name(cluster="Offset Values", "Trap 1X offset"=w1324, "Trap 2X offset"=w1325) -> (w1330:T14)
        n864 = Multiply(x=w1325, y=w1319) -> (x*y=w1323:dbl[])
        n865 = Subtract(x=w1324, y=w1323) -> (x-y=w1322:dbl[])
        n866 = local write "Offset Values"(w1330) -> ()
        n867 = case shown="True" "Auto read offset\ncorrection" {
          tunnel: w1322 -> [_ w1381]
          frame False {
          }
          frame True {
            n868 = property on="Setpoint offset\nCorrection values" class="Arr (strict)"("Val(Sgnl)"=w1381) -> ()  [unwired: 2 in, 2 out]
          }
        }
        n869 = property on="B factor" class="DigNum (strict)"("Val(Sgnl)"=w1319) -> ()  [unwired: 2 in, 2 out]
      }
      event "Symmetric Raster/Feedback?": Value Change {
        n870 = event-data() -> ()  [unwired: 7 out]
        n871 = xnode "Read/Write Control"("FPGA VI Reference In"=w1383, "Symmetric FB/Raster"="Symmetric Raster/Feedback?") -> ()  [unwired: 1 in, 2 out]
      }
      event "Abort MCL Scan": Value Change {
        n872 = event-data() -> ()  [unwired: 7 out]
        n873 = local write "MCL Scanning"(FALSE ("MCL Scanning")) -> ()
        n874 = xnode "Read/Write Control"("FPGA VI Reference In"=w1388, "error in"=w1387, "Abort scan (MCL)"="Abort MCL Scan") -> ("error out"=w1386:errorcluster)  [unwired: 1 out]
      }
      event "Update Count (MCL)": Value Change {
        n875 = event-data() -> ()  [unwired: 7 out]
        n876 = xnode "Read/Write Control"("FPGA VI Reference In"=w1392, "error in"=w1391, "MCL count"="Update Count (MCL)") -> ("error out"=w1390:errorcluster)  [unwired: 1 out]
      }
      event "Phase adjust (MCL)", "+ phase (MCL)", "- phase (MCL)": Value Change {
        n877 = event-data() -> ()  [unwired: 7 out]
        n878 = Negate(x="Phase adjust (MCL)") -> (-x=w1401:i16)
        n879 = Select(t=w1401, s="- phase (MCL)", f="Phase adjust (MCL)") -> (s? t:f=w1399:i16)
        n880 = Or(x="- phase (MCL)", y="+ phase (MCL)") -> (x .or. y?=w1394:bool)
        n881 = xnode "Read/Write Control"("FPGA VI Reference In"=w1403, "error in"=w1402, "Phase count adjustment (MCL)"=w1399) -> ("FPGA VI Reference Out"=w1395:T20, "error out"=w1396:errorcluster)
        n882 = xnode "Read/Write Control"("FPGA VI Reference In"=w1395, "error in"=w1396, "+ phase (MCL)"=w1394) -> ("error out"=w1393:errorcluster)  [unwired: 1 out]
      }
      event "Abort AOD Scan": Value Change {
        n883 = event-data() -> ()  [unwired: 7 out]
        n884 = flat-sequence {
          tunnel: w1408 -> [w1415]
          tunnel: w1407 -> [w1414]
          tunnel: [w1413] -> w1405
          tunnel: [w1409] -> w1404
          tunnel: [w1428] -> w1406
          tunnel: w1405 -> [w1428]
          tunnel: w1404 -> [w1427]
          frame #0 {
            n885 = local read "Save scans"() -> (w1411:bool)
            n886 = xnode "Read/Write Control"("FPGA VI Reference In"=w1415, "error in"=w1414, "Abort scan"="Abort AOD Scan") -> ("FPGA VI Reference Out"=w1409:T20, "error out"=w1413:errorcluster)
            n887 = local write "Raster Scanning..."(FALSE) -> ()
            n888 = case shown="True" w1411 {
              frame False {
              }
              frame True {
                n889 = local write "Stop Saving"(TRUE) -> ()
              }
            }
          }
          frame #1 {
            n890 = xnode "Read/Write Control"("FPGA VI Reference In"=w1427) -> ("BD1 Frequency Out 1"=w1418:u64)  [unwired: 1 in, 2 out]
            n891 = To Double Precision Float(number=w1418) -> (double precision float=w1424:dbl)
            n892 = Multiply(x=49125000.0, y=6.0) -> (x*y=w1423:dbl)
            n893 = Multiply(x=w1424, y=w1423) -> (x*y=w1421:dbl)
            n894 = Scale By Power Of 2(n=-48, x=w1421) -> (x*2^n=w1420:dbl)
            n895 = Divide(x=w1420, y=1000000.0) -> (x/y=w1417:dbl)
            n896 = property on="BD 1 Frequency 1 (MHz)" class="DigNum (strict)"("Val(Sgnl)"=w1417) -> ()  [unwired: 2 in, 2 out]
          }
        }
      }
      event "Continuous AOD Scanning": Value Change {
        n897 = event-data() -> ()  [unwired: 7 out]
        n898 = xnode "Read/Write Control"("FPGA VI Reference In"=w1432, "error in"=w1431, "Cont. Scan"="Continuous AOD Scanning") -> ("error out"=w1430:errorcluster)  [unwired: 1 out]
      }
      event "Index": Value Change {
        n899 = event-data() -> ()  [unwired: 7 out]
        n900 = call "Create new save file.vi"("Insert"="", "Ext"=".dat" ("string"), "Index In"="Index") -> ("Path Out"=→"Save file name":path, "Index Out"=w1433:dbl)
        "Save index" <- w1433
        n901 = local write "Index"(w1433) -> ()
      }
      event "AO1", "AO2": Value Change {
        w1448 = 10.0 ("y")
        w1447 = 32767.0 ("y")
        n902 = event-data() -> ()  [unwired: 7 out]
        n903 = local read "AO2"() -> (w1446:dbl)
        n904 = local read "AO1"() -> (w1443:dbl)
        n905 = Multiply(x=w1443, y=w1447) -> (x*y=w1442:dbl)
        n906 = Multiply(x=w1446, y=w1447) -> (x*y=w1445:dbl)
        n907 = Divide(x=w1442, y=w1448) -> (x/y=w1441:dbl)
        n908 = Divide(x=w1445, y=w1448) -> (x/y=w1444:dbl)
        n909 = To Word Integer(number=w1441) -> (16bit integer=w1449:i16)
        n910 = To Word Integer(number=w1444) -> (16bit integer=w1450:i16)
        n911 = xnode "Read/Write Control"("FPGA VI Reference In"=w1440, "error in"=w1439, "AO1 (Y)"=w1449, "AO2 (X)"=w1450) -> ("error out"=w1438:errorcluster)  [unwired: 1 out]
      }
      event "Inject Top:": Value Change {
        n912 = event-data() -> ()  [unwired: 7 out]
        n913 = disable-structure shown="Enabled" {
          disable-tunnel: "Inject Top:" -> [w1452 w1492]
          frame Disabled {
            n914 = local read "Chemyx Syringe Pump Serial Port"() -> (w1453:refnum<visa-resource-name>)
            n915 = local read "Pump write delay (ms)"() -> (w1454:dbl)
            n916 = case shown="True" w1452 {
              tunnel: w1454 -> [w1460 w1474]
              tunnel: w1453 -> [w1457 w1473]
              frame False {
                n917 = flat-sequence {
                  tunnel: w1457 -> [w1461]
                  tunnel: [w1461] -> w1458
                  tunnel: w1460 -> [_]
                  tunnel: [w1464] -> w1459
                  tunnel: w1458 -> [w1464]
                  tunnel: w1459 -> [w1465]
                  tunnel: [w1465] -> w1455
                  tunnel: [w1467] -> w1456
                  tunnel: w1455 -> [w1467]
                  tunnel: w1456 -> [w1469]
                  frame #0 {
                    n918 = call "Write to pump.vi"("string"="enter pump1", "VISA resource name"=w1461) -> ()  [unwired: 1 out]
                  }
                  frame #1 {
                    n919 = Wait (ms)(milliseconds to wait="Pump pause delay (ms)") -> ()  [unwired: 1 out]
                  }
                  frame #2 {
                    n920 = call "Write to pump.vi"("string"="stop", "VISA resource name"=w1465) -> ()  [unwired: 1 out]
                  }
                  frame #3 {
                    n921 = Wait (ms)(milliseconds to wait=u32 500) -> ()  [unwired: 1 out]
                  }
                  frame #4 {
                    n922 = call "Write to pump.vi"("string"="stop", "VISA resource name"=w1469) -> ()  [unwired: 1 out]
                  }
                }
              }
              frame True {
                n923 = flat-sequence {
                  tunnel: w1473 -> [w1483]
                  tunnel: w1474 -> [w1478]
                  tunnel: w1474 -> [w1485]
                  tunnel: w1473 -> [w1486]
                  tunnel: [w1486] -> w1471
                  tunnel: [w1488] -> w1472
                  tunnel: w1471 -> [w1488]
                  tunnel: w1472 -> [w1490]
                  frame #0 {
                    n924 = local read "All Pump Parameters"() -> (w1477:T6)
                    n925 = Unbundle By Name(w1477) -> ("Pump 1"=w1484:T33)
                    n926 = call "Set pump parameters.vi"("Pump write delay (ms)"=w1478, "Volume (uL)"="Ch 2 Inject Volume (uL)", "Rate (uL/h)"="Ch 1 Inject Rate (ul/h)", "Units"=4.0, "Pump #"=1.0, "Pump Parameters In"=w1484, "VISA resource name"=w1483) -> ("Pump Parameters Out"=w1476:T33)  [unwired: 3 in]
                    n927 = Bundle By Name(cluster=w1477, "Pump 1"=w1476) -> (w1475:T6)
                    n928 = local write "All Pump Parameters"(w1475) -> ()
                  }
                  frame #1 {
                    n929 = Wait (ms)(milliseconds to wait=w1485) -> ()  [unwired: 1 out]
                  }
                  frame #2 {
                    n930 = call "Write to pump.vi"("string"="start", "VISA resource name"=w1486) -> ()  [unwired: 1 out]
                  }
                  frame #3 {
                    n931 = Wait (ms)(milliseconds to wait=u32 500) -> ()  [unwired: 1 out]
                  }
                  frame #4 {
                    n932 = call "Write to pump.vi"("string"="start", "VISA resource name"=w1490) -> ()  [unwired: 1 out]
                  }
                }
              }
            }
          }
          frame Enabled {
            n933 = call "hamilton_controller.vi"("Open?"=w1492, "valve"=enum16{"A", "B", "C", "D", "ALL"}."B", "action"=T21."MOVE VALVE") -> ()  [unwired: 8 in, 1 out]
          }
        }
      }
      event "Main:": Value Change {
        n934 = event-data() -> ()  [unwired: 7 out]
        n935 = disable-structure shown="Enabled" {
          disable-tunnel: "Main:" -> [_ w1536]
          frame Disabled {
            n936 = local read "Pump write delay (ms)"() -> (w1497:dbl)
            n937 = case shown="False" w1498 {
              tunnel: w1497 -> [w1504 w1518]
              tunnel: "Chemyx Syringe Pump Serial Port" -> [w1501 w1517]
              frame False {
                n938 = flat-sequence {
                  tunnel: w1501 -> [w1505]
                  tunnel: [w1505] -> w1502
                  tunnel: w1504 -> [_]
                  tunnel: [w1508] -> w1503
                  tunnel: w1502 -> [w1508]
                  tunnel: w1503 -> [w1509]
                  tunnel: [w1509] -> w1499
                  tunnel: [w1511] -> w1500
                  tunnel: w1499 -> [w1511]
                  tunnel: w1500 -> [w1513]
                  frame #0 {
                    n939 = call "Write to pump.vi"("string"="enter pump3", "VISA resource name"=w1505) -> ()  [unwired: 1 out]
                  }
                  frame #1 {
                    n940 = local read "Pump pause delay (ms)"() -> (w1507:u32)
                    n941 = Wait (ms)(milliseconds to wait=w1507) -> ()  [unwired: 1 out]
                  }
                  frame #2 {
                    n942 = call "Write to pump.vi"("string"="stop", "VISA resource name"=w1509) -> ()  [unwired: 1 out]
                  }
                  frame #3 {
                    n943 = Wait (ms)(milliseconds to wait=u32 0) -> ()  [unwired: 1 out]
                  }
                  frame #4 {
                    n944 = call "Write to pump.vi"("string"="stop", "VISA resource name"=w1513) -> ()  [unwired: 1 out]
                  }
                }
              }
              frame True {
                n945 = flat-sequence {
                  tunnel: w1517 -> [w1527]
                  tunnel: w1518 -> [w1522]
                  tunnel: w1518 -> [w1529]
                  tunnel: w1517 -> [w1530]
                  tunnel: [w1530] -> w1515
                  tunnel: [w1533] -> w1516
                  tunnel: w1515 -> [w1533]
                  tunnel: w1516 -> [w1534]
                  frame #0 {
                    n946 = local read "All Pump Parameters"() -> (w1521:T6)
                    n947 = Unbundle By Name(w1521) -> ("Pump 3"=w1528:T33)
                    n948 = call "Set pump parameters.vi"("Pump write delay (ms)"=w1522, "Volume (uL)"="Ch 3 Inject Volume (uL)", "Rate (uL/h)"="Ch 3 Inject Rate (ul/h)", "Units"=4.0, "Pump #"=3.0, "Pump Parameters In"=w1528, "VISA resource name"=w1527) -> ("Pump Parameters Out"=w1520:T33)  [unwired: 3 in]
                    n949 = Bundle By Name(cluster=w1521, "Pump 3"=w1520) -> (w1519:T6)
                    n950 = local write "All Pump Parameters"(w1519) -> ()
                  }
                  frame #1 {
                    n951 = Wait (ms)(milliseconds to wait=w1529) -> ()  [unwired: 1 out]
                  }
                  frame #2 {
